vi "Add.vi"(8 "error in (no error)":errorcluster caption="错误输入（无错误）", 11 "Point 输入":refnum<class "Point.lvclass"> caption="DNL_LabVIEW Object in") -> (0 "error out":errorcluster caption="错误输出", 3 "Point 输出":refnum<class "Point.lvclass"> caption="DNL_LabVIEW Object out")   [LabVIEW 2011, in "Point.lvclass"]
uses:
  Point.lvclass
panel:
  in  "Point 输入":refnum<class "Point.lvclass"> caption="DNL_LabVIEW Object in"
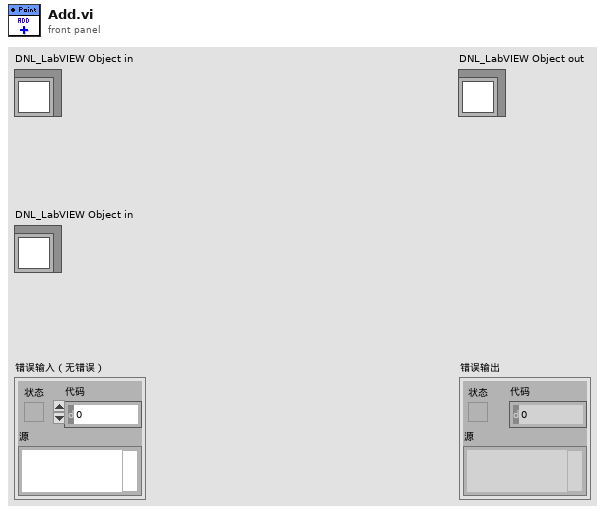
[diagram p1: front panel]
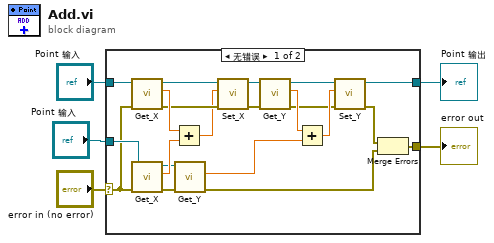
[diagram p0: block diagram]
diagram:
  n1 = case shown="无错误" "error in (no error)" {
    selector: "error in (no error)" -> [w24 w28]
    tunnel: [w6 w28] -> w4
    tunnel: [w9 w27] -> w2
    tunnel: "Point 输入" -> [w26 w27]
    tunnel: "Point 输入" -> [w25 _]
    frame No Error {
      n2 = call "Get_X.vi"("error in (no error)"=w24, "Point输入"=w26) -> ("error out"=w21:errorcluster, "X"=w22:dbl, "Point输出"=w20:refnum<class "Point.lvclass">)  [unwired: 7 in]
      n3 = call "Get_X.vi"("error in (no error)"=w24, "Point输入"=w25) -> ("error out"=w17:errorcluster, "X"=w23:dbl, "Point输出"=w18:refnum<class "Point.lvclass">)  [unwired: 7 in]
      n4 = Add(x=w22, y=w23) -> (x+y=w19:dbl)
      n5 = call "Get_Y.vi"("error in (no error)"=w17, "Point输入"=w18) -> ("error out"=w7:errorcluster, "Y"=w13:dbl)  [unwired: 7 in, 1 out]
      n6 = call "Set_X.vi"("error in (no error)"=w21, "X"=w19, "Point输入"=w20) -> ("error out"=w15:errorcluster, "Point输出"=w16:refnum<class "Point.lvclass">)  [unwired: 7 in]
      n7 = call "Get_Y.vi"("error in (no error)"=w15, "Point输入"=w16) -> ("error out"=w10:errorcluster, "Y"=w14:dbl, "Point输出"=w11:refnum<class "Point.lvclass">)  [unwired: 7 in]
      n8 = Add(x=w14, y=w13) -> (x+y=w12:dbl)
      n9 = call "Set_Y.vi"("error in (no error)"=w10, "Y"=w12, "Point输入"=w11) -> ("error out"=w8:errorcluster, "Point输出"=w9:refnum<class "Point.lvclass">)  [unwired: 7 in]
      n10 = Merge Errors(w8, w7) -> (w6:errorcluster)
    }
    frame Error {
    }
  }
  "error out" <- w4
  "Point 输出" <- w2
